vi "MM6.InitDiscArchiver.vi"(0 "i ref in":refnum<vi>, 3 "ms timeout (10000)":i32=10000, 5 "error in (no error)":errorcluster) -> (14 "i ref out":refnum<vi>, 17 "timed out":bool, 19 "error out":errorcluster)   [LabVIEW 2014, in "MM6.lvlib"]
doc: "Initializes the disc archiver."
uses:
  MM6.lvlib
  CSCore/CSSystem/CoreLib/CoreLib.short 2 byte array.vi
  CSCore/CSSystem/CoreLib/CoreLib.string 2 byte array.vi
  CSCore/CSSystem/CoreLib/CoreLib.lvlib
  CSCore/BaseProcess/BaseProcess.lvlib
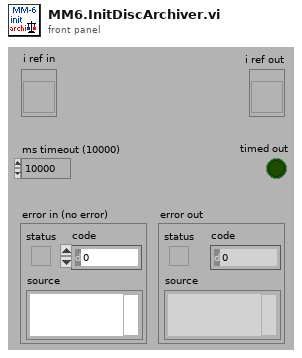
[diagram p1: front panel]
types:
  T1 = typedef "CoreDefs.rawDataType.ctl" = i8[]
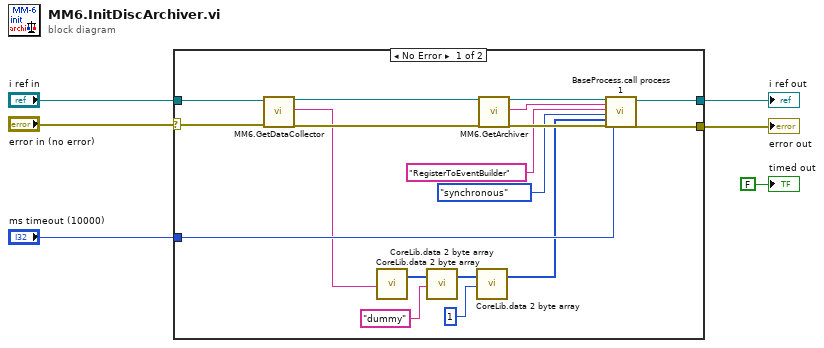
[diagram p0: block diagram]
diagram:
  n1 = case shown="No Error" "error in (no error)" {
    selector: "error in (no error)" -> [w16 w25]
    tunnel: "i ref in" -> [w21 w26]
    tunnel: [w20 w25] -> w4
    tunnel: [w19 w26] -> w3
    tunnel: "ms timeout (10000)" -> [w17 _]
    frame No Error {
      n2 = call "MM6.GetDataCollector.vi"("i ref in"=w21, "error in (no error)"=w16) -> ("i ref out"=w23:refnum<vi>, "data collector"=w14:string, "error out"=w22:errorcluster)  [unwired: 15 in]
      n3 = call-poly "CoreLib.data 2 byte array.vi"("string"=w14) -> ("byteArray out"=w15:T1)  [unwired: 18 in]
      n4 = call-poly "CoreLib.data 2 byte array.vi"("byteArray"=w15, "string"="dummy") -> ("byteArray out"=w18:T1)  [unwired: 17 in]
      n5 = call-poly "CoreLib.data 2 byte array.vi"("byteArray"=w18, "i16"=i16 1) -> ("byteArray out"=w8:T1)  [unwired: 17 in]
      n6 = call "MM6.GetArchiver.vi"("i ref in"=w23, "error in (no error)"=w22) -> ("i ref out"=w24:refnum<vi>, "archiver"=w12:string, "error out"=w11:errorcluster)  [unwired: 15 in]
      n7 = call "BaseProcess.call process 1.vi"("i ref in"=w24, "Object"=w12, "Selector"="RegisterToEventBuilder", "CallType"=enum16{"simple", "synchronous", "asynchronous"}."synchronous", "Data"=w8, "error in (no error)"=w11, "timeout (ms)"=w17) -> ("i ref out"=w19:refnum<vi>, "error out"=w20:errorcluster)  [unwired: 10 in, 1 out]
    }
    frame Error {
    }
  }
  "error out" <- w4
  "i ref out" <- w3
  "timed out" <- FALSE ("timed out")
